vi "Read Saving RDs.vi"(8 "error in (no error)":errorcluster, 11 "CRDS in":refnum<class "CRDS.lvclass">) -> (0 "error out":errorcluster, 2 "Saving RDs":bool, 3 "CRDS out":refnum<class "CRDS.lvclass">)   [LabVIEW 2016, in "CRDS Lib.lvlib" / "CRDS.lvclass"]
uses:
  CRDS.lvclass
  CRDS.lvclass/CRDS.ctl
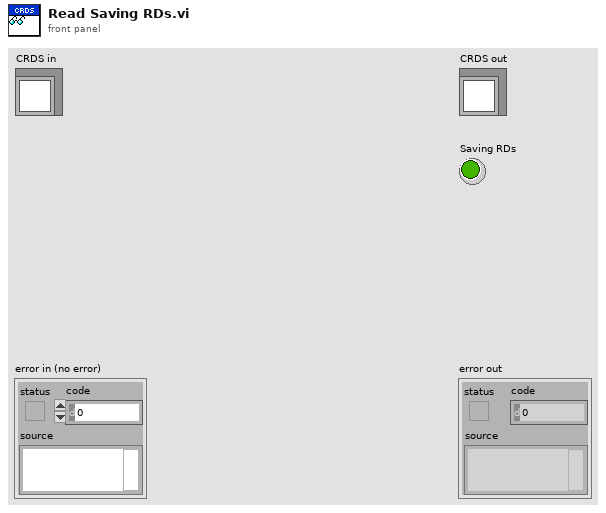
[diagram p1: front panel]
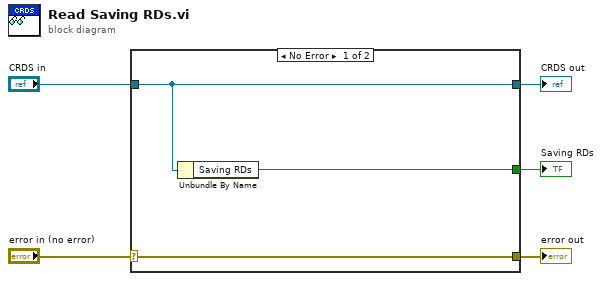
[diagram p0: block diagram]
diagram:
  n1 = case shown="No Error" "error in (no error)" {
    selector: "error in (no error)" -> [w8 w9]
    tunnel: [w8 w9] -> w4
    tunnel: [w7 w10] -> w2
    tunnel: "CRDS in" -> [w7 w10]
    tunnel: [w6 _] -> w1
    frame No Error {
      n2 = Unbundle By Name(w7) -> ("Saving RDs"=w6:bool)
    }
    frame Error {
    }
  }
  "error out" <- w4
  "CRDS out" <- w2
  "Saving RDs" <- w1
